vi "Start Log.vi"(8 "error in (no error)":errorcluster, 10 "tdms file":refnum<k34>, 11 "Acquired Result in":refnum<class "Acquired Result.lvclass">) -> (0 "error out":errorcluster, 2 "tdms file out":refnum<k34>, 3 "Acquired Result out":refnum<class "Acquired Result.lvclass">)   [LabVIEW 2016, in "Acquired Result.lvclass"]
uses:
  Acquired Result.lvclass
  Acquired Result.lvclass/Acquired Result.ctl
  Read Group.vi
  Read Channels.vi
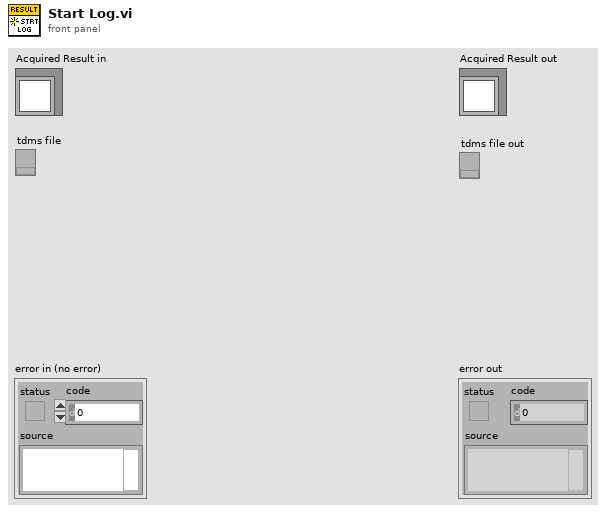
[diagram p1: front panel]
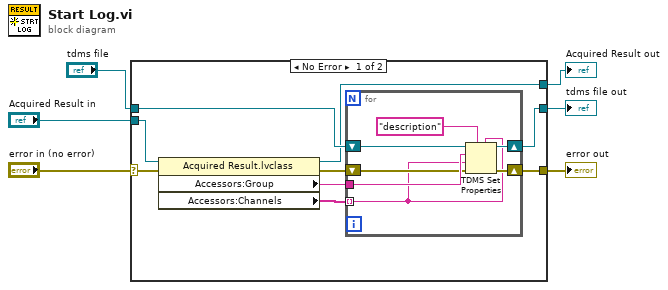
[diagram p0: block diagram]
diagram:
  n1 = case shown="No Error" "error in (no error)" {
    selector: "error in (no error)" -> [w8 w25]
    tunnel: [w14 w25] -> w5
    tunnel: [w9 w24] -> w3
    tunnel: "Acquired Result in" -> [w10 w24]
    tunnel: "tdms file" -> [w12 w23]
    tunnel: [w11 w23] -> w1
    frame No Error {
      n2 = property class="Acquired Result.lvclass"(reference=w10, error in=w8) -> (reference out=w9:refnum<class "Acquired Result.lvclass">, error out=w7:errorcluster, "Accessors:Group"=w15:string, "Accessors:Channels"=w13:string[])
      n3 = for {
        tunnel: w15 -> [w20]
        shift-right: [w21] -> w11
        shift-left: w12 -> [w22]
        shift-right: [w18] -> w14
        shift-left: w7 -> [w19]
        tunnel: w13 -> [w16] mode=indexing
        n4 = TDMS Set Properties(5:w16, 7:"description", 8:w19, 9:w16, 10:w20, 11:w22) -> (0:w18:errorcluster, 3:w21:refnum<k34>)  [unwired: 2 out]
      }
    }
    frame Error {
    }
  }
  "error out" <- w5
  "Acquired Result out" <- w3
  "tdms file out" <- w1
